vi "kvCanGetChannelDataChannelName.vi"(2 "error in (no error)":errorcluster, 3 "Channel Number":i32) -> (0 "error out":errorcluster, 1 "Channel Name":string)   [LabVIEW 2022 SP3]
doc: "Get the clear-text name of the channel."
uses:
  canlib32.dll
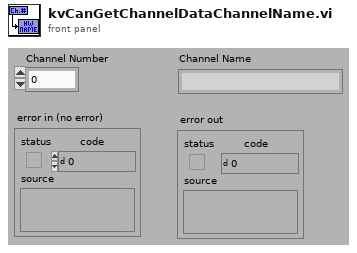
[diagram p1: front panel]
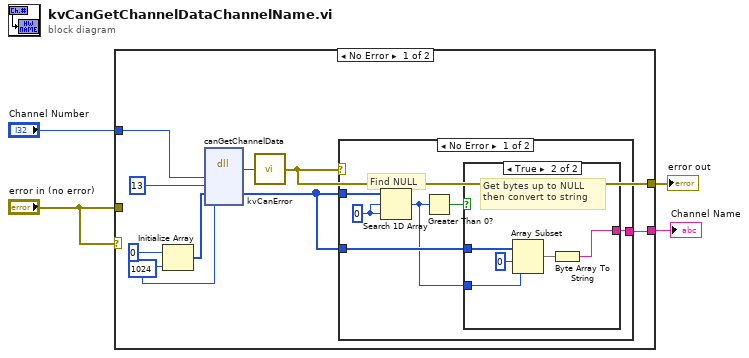
[diagram p0: block diagram]
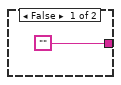
[diagram p2: hidden frame]
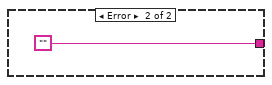
[diagram p3: hidden frame]
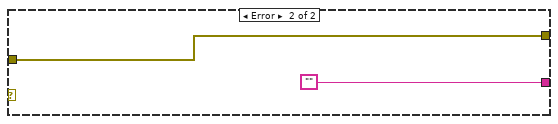
[diagram p4: hidden frame]
diagram:
  n1 = case shown="No Error" "error in (no error)" {
    tunnel: "error in (no error)" -> [_ w28]
    tunnel: [w11 w28] -> w3
    tunnel: "Channel Number" -> [w13 _]
    tunnel: [w6 ""] -> w1
    frame No Error {
      w10 = 1024
      n2 = Initialize Array(u8 0, w10) -> (w8:u8[])
      n3 = dll-call lib="canlib32.dll" fn="canGetChannelData" label="Call canGetChannelData"("channel"=w13, "item"=13, "buffer"=w8, "bufsize"=w10) -> (w12:i32, "buffer"=w5:u8[])  [unwired: 6 in, 2 out]
      n4 = call "kvCanError.vi"("error code"=w12) -> ("error out"=w11:errorcluster)
      n5 = case shown="No Error" w11 {
        tunnel: [w16 ""] -> w6
        tunnel: w5 -> [w18 _]
        tunnel: w5 -> [w15 _]
        frame No Error {
          w19 = 0
          # "Find NULL"
          n6 = Search 1D Array(1D array=w18, element=w19, start index (0)=w19) -> (index of element=w14:i32)
          n7 = Greater Than 0?(x=w14) -> (x > 0?=w17:bool)
          n8 = case shown="True" w17 {
            tunnel: ["" w21] -> w16
            tunnel: w15 -> [_ w23]
            tunnel: w14 -> [_ w22]
            frame False {
            }
            frame True {
              # "Get bytes up to NULL\nthen convert to string"
              n9 = Array Subset(array=w23, index=0, length=w22) -> (w24:u8[])
              n10 = Byte Array To String(unsigned byte array=w24) -> (string=w21:string)
            }
          }
        }
        frame Error {
        }
      }
    }
    frame Error {
    }
  }
  "error out" <- w3
  "Channel Name" <- w1
